vi "Robot State.vi"() -> ()   [LabVIEW 2019]
uses:
  Controls/Robot State.ctl
  Controls/Robot Pivot Motion Commands.ctl
  Controls/Pivot Motor Commands.ctl
  Controls/Robot Drive Mode.ctl
  Controls/Enable Actions.ctl
  Controls/Lift System Actions.ctl
  Controls/Spinner Actions.ctl
  Controls/Ball System Actions.ctl
panel:
  out "Robot State":T1
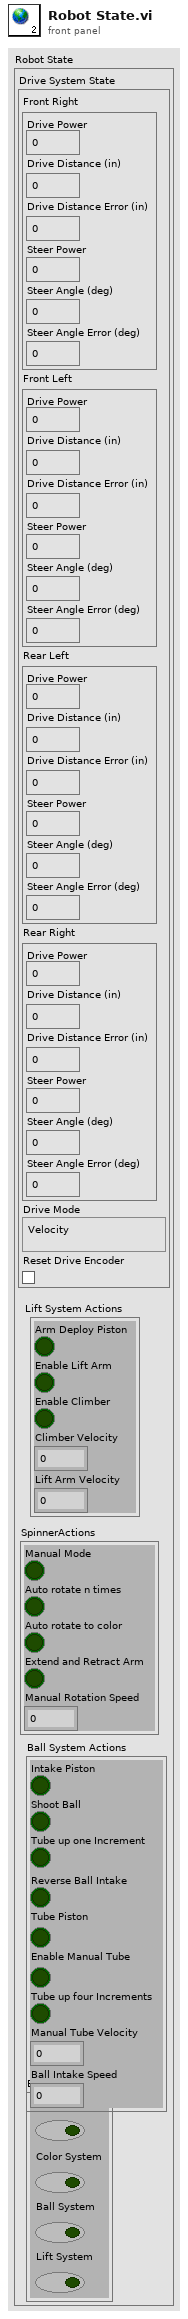
[diagram p1: front panel]
types:
  T1 = typedef "Robot State.ctl" = cluster{"Drive System State":T2, "Enable Actions":T5, "Lift System Actions":T6, "SpinnerActions":T7, "Ball System Actions":T8}
  T2 = typedef "Robot Pivot Motion Commands.ctl" = cluster{"Front Right":T3, "Front Left":T3, "Rear Left":T3, "Rear Right":T3, "Drive Mode":T4, "Reset Drive Encoder":bool}
  T3 = typedef "Pivot Motor Commands.ctl" = cluster{"Drive Power":dbl, "Drive Distance (in)":dbl, "Drive Distance Error (in)":dbl, "Steer Power":dbl, "Steer Angle (deg)":dbl, "Steer Angle Error (deg)":dbl}
  T4 = typedef "Robot Drive Mode.ctl" = enum16{"Velocity", "Distance"}
  T5 = typedef "Enable Actions.ctl" = cluster{"Swerve Drive":bool, "Color System":bool, "Ball System":bool, "Lift System":bool}
  T6 = typedef "Lift System Actions.ctl" = cluster{"Arm Deploy Piston":bool, "Enable Lift Arm":bool, "Enable Climber":bool, "Climber Velocity":dbl, "Lift Arm Velocity":dbl}
  T7 = typedef "Spinner Actions.ctl" = cluster{"Manual Mode ":bool, "Auto rotate n times":bool, "Auto rotate to color\t":bool, "Extend and Retract Arm\t":bool, "Manual Rotation Speed":dbl}
  T8 = typedef "Ball System Actions.ctl" = cluster{"Intake Piston ":bool, "Shoot Ball":bool, "Tube up one Increment\t":bool, "Reverse Ball Intake":bool, "Tube Piston":bool, "Enable Manual Tube":bool, "Tube up four Increments":bool, "Manual Tube Velocity":dbl, "Ball Intake Speed":dbl}
diagram:
